vi "Plot Phase.vi"(8 "Target Lossy Data":T2) -> (3 "Phase Waveform":T1)   [LabVIEW 2018]
uses:
  Target Lossy Data.ctl
  Sensor Data.ctl
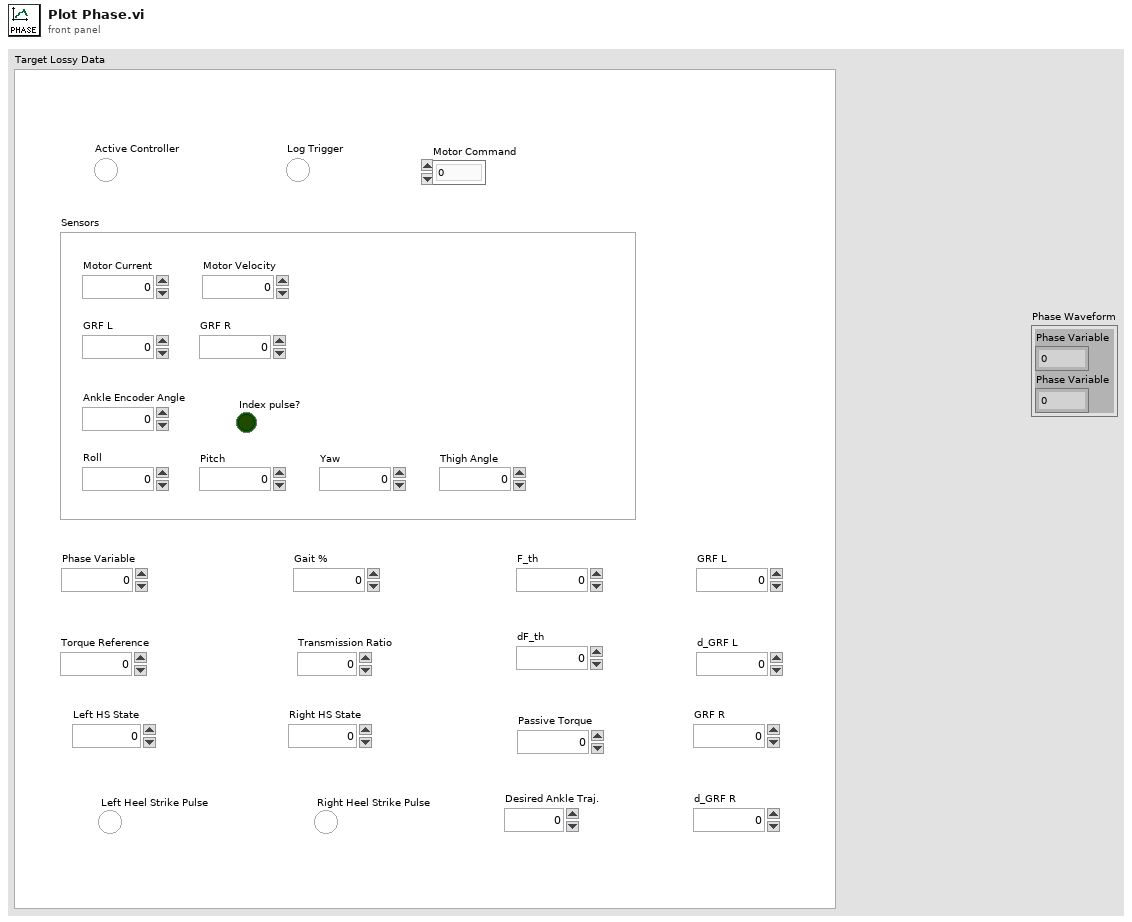
[diagram p1: front panel]
types:
  T1 = cluster{"Phase Variable":dbl, "Phase Variable":dbl}
  T2 = typedef "Target Lossy Data.ctl" = cluster{"Active Controller":bool, "Log Trigger":bool, "Sensors":T3, "Motor Command":dbl, "Phase Variable":dbl, "Left HS State":u32, "Left Heel Strike Pulse":bool, "Gait %":dbl, "Torque Reference":dbl, "Passive Torque":dbl, "F_th":dbl, "dF_th":dbl, "d_GRF L":dbl, "GRF L":dbl, "Transmission Ratio":dbl, "Desired Ankle Traj.":dbl, "Right HS State":u32, "Right Heel Strike Pulse":bool, "d_GRF R":dbl, "GRF R":dbl}
  T3 = typedef "Sensor Data.ctl" = cluster{"Motor Current":dbl, "Motor Velocity":dbl, "Ankle Encoder Angle":dbl, "GRF L":dbl, "GRF R":dbl, "Index pulse?":bool, "Roll":dbl, "Pitch":dbl, "Yaw":dbl, "Thigh Angle":dbl}
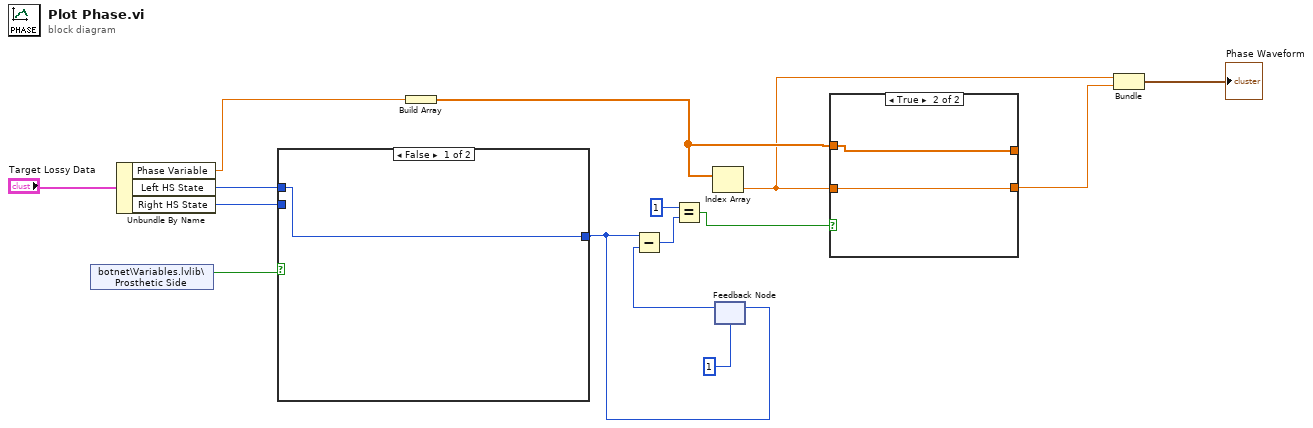
[diagram p0: block diagram]
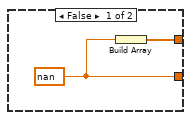
[diagram p2: hidden frame]
diagram:
  n1 = shared-variable "botnet\\Variables.lvlib\\Prosthetic Side"() -> (w14:bool)  [unwired: 1 in, 1 out]
  n2 = Unbundle By Name("Target Lossy Data") -> ("Phase Variable"=w11:dbl, "Left HS State"=w12:u32, "Right HS State"=w13:u32)
  n3 = case shown="False" w14 {
    tunnel: w13 -> [_ w17]
    tunnel: w12 -> [w16 _]
    tunnel: [w16 w17] -> w6
    frame False {
    }
    frame True {
    }
  }
  n4 = Build Array(w11) -> (w4:dbl[])
  n5 = Index Array(array=w4) -> (element=w2:dbl)  [unwired: 1 in]
  n6 = feedback #1(1) -> (w9:u32)
  n7 = Subtract(x=w6, y=w9) -> (x-y=w7:u32)
  n8 = Equal?(x=1, y=w7) -> (x = y?=w5:bool)
  n9 = feedback-in #1(w6) -> ()
  n10 = case shown="True" w5 {
    tunnel: w2 -> [_ w20]
    tunnel: w4 -> [_ w21]
    tunnel: [w19 w21] -> _
    tunnel: [w18 w20] -> w3
    frame False {
      w18 = nan
      n11 = Build Array(w18) -> (w19:dbl[])
    }
    frame True {
    }
  }
  n12 = Bundle("Phase Variable"=w2, "Phase Variable"=w3) -> (→"Phase Waveform":T1)  [unwired: 1 in]
